vi "CSS validation.vi"() -> ()   [LabVIEW 2014]
uses:
  <vilib>/Utility/file.llb/Read From Spreadsheet File (string).vi
  <vilib>/Utility/file.llb/Write To Spreadsheet File (string).vi
panel:
  in  "cluster centers":string[](array[string])=["1 0 -1 1 -1 0 -4 1 -4 0 1", "2 0 -1 2 -1 0 -2 2 -2 0 2", "3 0 -3 3 -3 0 -2 3 -2 0 3", "4 0 -3 4 -3 0 -4 4 -4 0 4", "-1 1 -4 0 -4 4 -3 4 -4 0 -4 1 -1", "-1 2 -2 0 -2 3 -3 3 -2 0 -2 2 -1", "-4 1 -1 0 -1 2 -2 2 -1 0 -1 1 -4", "-4 4 -3 0 -3 3 -2 3 -3 0 -3 4 -4", "0 -4 1 -1 0 -3 3 -2 3 -3 0 -1 1 -4 0", "0 -4 4 -3 0 -1 2 -2 2 -1 0 -3 4 -4 0"]
  in  "cluster centers (original) 4":string[](array[string])=["0 -1 1 -4 0 -4 1 -1 0", "0 -1 2 -2 0 -2 2 -1 0", "0 -2 3 -3 0 -3 3 -2 0", "0 -3 4 -4 0 -4 4 -3 0", "0 -1 1 -4 4 -3 0 -3 4 -4 1 -1 0", "0 -1 2 -2 3 -3 0 -3 3 -2 2 -1 0", "0 -4 1 -1 2 -2 0 -2 2 -1 1 -4 0", "0 -4 4 -3 3 -2 0 -2 3 -3 4 -4 0", "0 -1 1 -4 0 -2 3 -3 0 -3 3 -2 0 -4 1 -1 0", "0 -1 2 -2 0 -4 4 -3 0 -3 4 -4 0 -2 2 -1 0"]
  in  "cluster centers 3":string[](array[string])=["0 -1 1 0 1 -4 0 -4 1 0 1 -1 0 -1 1 0 1 -4 0 -4 1 0 1 -1 0 -1 1 0 1 -4 0 -4 1 0 1 -1 0", "0 -1 2 0 2 -2 0 -2 2 0 2 -1 0 -1 2 0 2 -2 0 -2 2 0 2 -1 0 -1 2 0 2 -2 0 -2 2 0 2 -1 0", "0 -2 3 0 3 -3 0 -3 3 0 3 -2 0 -2 3 0 3 -3 0 -3 3 0 3 -2 0 -2 3 0 3 -3 0 -3 3 0 3 -2 0", "0 -3 4 0 4 -4 0 -4 4 0 4 -3 0 -3 4 0 4 -4 0 -4 4 0 4 -3 0 -3 4 0 4 -4 0 -4 4 0 4 -3 0", "0 -1 1 -4 0 -4 4 -3 0 -3 4 -4 0 -4 1 -1 0 0 -1 1 -4 0 -4 4 -3 0 -3 4 -4 0 -4 1 -1 0 0 -1 1 -4 0 -4 4 -3 0 -3 4 -4 0 -4 1 -1 0", "0 -1 2 -2 0 -2 3 -3 0 -3 3 -2 0 -2 2 -1 0 0 -1 2 -2 0 -2 3 -3 0 -3 3 -2 0 -2 2 -1 0 0 -1 2 -2 0 -2 3 -3 0 -3 3 -2 0 -2 2 -1 0", "0 -4 1 -1 0 -1 2 -2 0 -2 2 -1 0 -1 1 -4 0 0 -4 1 -1 0 -1 2 -2 0 -2 2 -1 0 -1 1 -4 0 0 -4 1 -1 0 -1 2 -2 0 -2 2 -1 0 -1 1 -4 0", "0 -4 4 -3 0 -3 3 -2 0 -2 3 -3 0 -3 4 -4 0 0 -4 4 -3 0 -3 3 -2 0 -2 3 -3 0 -3 4 -4 0 0 -4 4 -3 0 -3 3 -2 0 -2 3 -3 0 -3 4 -4 0", "0 -1 1 -4 0 -4 1 -1 0 -3 3 -2 0 -2 3 -3 0 -1 1 -4 0 -4 1 -1 0 -3 3 -2 0 -2 3 -3 0 -1 1 -4 0 -4 1 -1 0 -3 3 -2 0 -2 3 -3 0", "0 -4 4 -3 0 -3 4 -4 0 -2 2 -1 0 -1 2 -2 0 -4 4 -3 0 -3 4 -4 0 -2 2 -1 0 -1 2 -2 0 -4 4 -3 0 -3 4 -4 0 -2 2 -1 0 -1 2 -2 0"]
  out "size(s)":i32
  in  "cluster centers (original) 3":string[](array[string])=["0 -1 1 -4 0 -4 1 -1 0 -1 1 -4 0 -4 1 -1 0 -1 1 -4 0 -4 1 -1 0", "0 -1 2 -2 0 -2 2 -1 0 -1 2 -2 0 -2 2 -1 0 -1 2 -2 0 -2 2 -1 0", "0 -2 3 -3 0 -3 3 -2 0 -2 3 -3 0 -3 3 -2 0 -2 3 -3 0 -3 3 -2 0", "0 -3 4 -4 0 -4 4 -3 0 -3 4 -4 0 -4 4 -3 0 -3 4 -4 0 -4 4 -3 0", "0 -1 1 -4 4 -3 0 -3 4 -4 1 -1 0 -1 1 -4 4 -3 0 -3 4 -4 1 -1 0 -1 1 -4 4 -3 0 -3 4 -4 1 -1 0", "0 -1 2 -2 3 -3 0 -3 3 -2 2 -1 0 -1 2 -2 3 -3 0 -3 3 -2 2 -1 0 -1 2 -2 3 -3 0 -3 3 -2 2 -1 0", "0 -4 1 -1 2 -2 0 -2 2 -1 1 -4 0 -4 1 -1 2 -2 0 -2 2 -1 1 -4 0 -4 1 -1 2 -2 0 -2 2 -1 1 -4 0", "0 -4 4 -3 3 -2 0 -2 3 -3 4 -4 0 -4 4 -3 3 -2 0 -2 3 -3 4 -4 0 -4 4 -3 3 -2 0 -2 3 -3 4 -4 0", "0 -1 1 -4 0 -2 3 -3 0 -3 3 -2 0 -4 1 -1 0 -1 1 -4 0 -2 3 -3 0 -3 3 -2 0 -4 1 -1 0 -1 1 -4 0 -2 3 -3 0 -3 3 -2 0 -4 1 -1 0", "0 -1 2 -2 0 -4 4 -3 0 -3 4 -4 0 -2 2 -1 0 -1 2 -2 0 -4 4 -3 0 -3 4 -4 0 -2 2 -1 0 -1 2 -2 0 -4 4 -3 0 -3 4 -4 0 -2 2 -1 0"]
  in  "cluster centers (original) 2":string[](array[string])=["0 -1 1 -4 0 -4 1 -1 0", "0 -1 2 -2 0 -2 2 -1 0", "0 -2 3 -3 0 -3 3 -2 0", "0 -3 4 -4 0 -4 4 -3 0", "0 -1 1 -4 4 -3 0 -3 4 -4 1 -1 0", "0 -1 2 -2 3 -3 0 -3 3 -2 2 -1 0", "0 -4 1 -1 2 -2 0 -2 2 -1 1 -4 0", "0 -4 4 -3 3 -2 0 -2 3 -3 4 -4 0", "0 -1 1 -4 0 -2 3 -3 0 -3 3 -2 0 -4 1 -1 0", "0 -1 2 -2 0 -4 4 -3 0 -3 4 -4 0 -2 2 -1 0"]
  out "results":string[][](array[string])
  in  "cluster centers 2 centers for diagonals - long - original clusters 5":string[](array[string])=["1 0 -1 1 -1 0 -4 1 -4 0 1 0 -1 1 -1 0 -4 1 -4 0 1 0 -1 1 -1 0 -4 1 -4 0 1 0 -1 1 -1 0 -4 1 -4 0 1 0 -1 1 -1 0 -4 1 -4 0 1", "2 0 -1 2 -1 0 -2 2 -2 0 2 0 -1 2 -1 0 -2 2 -2 0 2 0 -1 2 -1 0 -2 2 -2 0 2 0 -1 2 -1 0 -2 2 -2 0 2 0 -1 2 -1 0 -2 2 -2 0 2", "3 0 -3 3 -3 0 -2 3 -2 0 3 0 -3 3 -3 0 -2 3 -2 0 3 0 -3 3 -3 0 -2 3 -2 0 3 0 -3 3 -3 0 -2 3 -2 0 3 0 -3 3 -3 0 -2 3 -2 0 3", "4 0 -3 4 -3 0 -4 4 -4 0 4 0 -3 4 -3 0 -4 4 -4 0 4 0 -3 4 -3 0 -4 4 -4 0 4 0 -3 4 -3 0 -4 4 -4 0 4 0 -3 4 -3 0 -4 4 -4 0 4", "-1 1 -4 0 -4 4 -3 4 -4 0 -4 1 -1 1 -4 0 -4 4 -3 4 -4 0 -4 1 -1 1 -4 0 -4 4 -3 4 -4 0 -4 1 -1 1 -4 0 -4 4 -3 4 -4 0 -4 1 -1 1 -4 0 -4 4 -3 4 -4 0 -4 1 -1", "-1 2 -2 0 -2 3 -3 3 -2 0 -2 2 -1 2 -2 0 -2 3 -3 3 -2 0 -2 2 -1 2 -2 0 -2 3 -3 3 -2 0 -2 2 -1 2 -2 0 -2 3 -3 3 -2 0 -2 2 -1 2 -2 0 -2 3 -3 3 -2 0 -2 2 -1", "-4 1 -1 0 -1 2 -2 2 -1 0 -1 1 -4 1 -1 0 -1 2 -2 2 -1 0 -1 1 -4 1 -1 0 -1 2 -2 2 -1 0 -1 1 -4 1 -1 0 -1 2 -2 2 -1 0 -1 1 -4 1 -1 0 -1 2 -2 2 -1 0 -1 1 -4", "-4 4 -3 0 -3 3 -2 3 -3 0 -3 4 -4 4 -3 0 -3 3 -2 3 -3 0 -3 4 -4 4 -3 0 -3 3 -2 3 -3 0 -3 4 -4 4 -3 0 -3 3 -2 3 -3 0 -3 4 -4 4 -3 0 -3 3 -2 3 -3 0 -3 4 -4", "0 1 -1 0 -3 3 0 3 -3 0 -1 1 0 1 -1 0 -3 3 0 3 -3 0 -1 1 0 1 -1 0 -3 3 0 3 -3 0 -1 1 0 1 -1 0 -3 3 0 3 -3 0 -1 1 0 1 -1 0 -3 3 0 3 -3 0 -1 1 0", "0 1 -4 0 -2 3 0 3 -2 0 -4 1 0 1 -4 0 -2 3 0 3 -2 0 -4 1 0 1 -4 0 -2 3 0 3 -2 0 -4 1 0 1 -4 0 -2 3 0 3 -2 0 -4 1 0 1 -4 0 -2 3 0 3 -2 0 -4 1 0", "0 4 -3 0 -1 2 0 2 -1 0 -3 4 0 4 -3 0 -1 2 0 2 -1 0 -3 4 0 4 -3 0 -1 2 0 2 -1 0 -3 4 0 4 -3 0 -1 2 0 2 -1 0 -3 4 0 4 -3 0 -1 2 0 2 -1 0 -3 4 0", "0 4 -4 0 -2 2 0 2 -2 0 -4 4 0 4 -4 0 -2 2 0 2 -2 0 -4 4 0 4 -4 0 -2 2 0 2 -2 0 -4 4 0 4 -4 0 -2 2 0 2 -2 0 -4 4 0 4 -4 0 -2 2 0 2 -2 0 -4 4 0"]
  in  "cluster centers 2 centers for diagonals - long - original clusters 4":string[](array[string])=["1 0 -1 1 -1 0 -4 1 -4 0 1 0 -1 1 -1 0 -4 1 -4 0 1 0 -1 1 -1 0 -4 1 -4 0 1 0 -1 1 -1 0 -4 1 -4 0 1", "2 0 -1 2 -1 0 -2 2 -2 0 2 0 -1 2 -1 0 -2 2 -2 0 2 0 -1 2 -1 0 -2 2 -2 0 2 0 -1 2 -1 0 -2 2 -2 0 2", "3 0 -3 3 -3 0 -2 3 -2 0 3 0 -3 3 -3 0 -2 3 -2 0 3 0 -3 3 -3 0 -2 3 -2 0 3 0 -3 3 -3 0 -2 3 -2 0 3", "4 0 -3 4 -3 0 -4 4 -4 0 4 0 -3 4 -3 0 -4 4 -4 0 4 0 -3 4 -3 0 -4 4 -4 0 4 0 -3 4 -3 0 -4 4 -4 0 4", "-1 1 -4 0 -4 4 -3 4 -4 0 -4 1 -1 1 -4 0 -4 4 -3 4 -4 0 -4 1 -1 1 -4 0 -4 4 -3 4 -4 0 -4 1 -1 1 -4 0 -4 4 -3 4 -4 0 -4 1 -1", "-1 2 -2 0 -2 3 -3 3 -2 0 -2 2 -1 2 -2 0 -2 3 -3 3 -2 0 -2 2 -1 2 -2 0 -2 3 -3 3 -2 0 -2 2 -1 2 -2 0 -2 3 -3 3 -2 0 -2 2 -1", "-4 1 -1 0 -1 2 -2 2 -1 0 -1 1 -4 1 -1 0 -1 2 -2 2 -1 0 -1 1 -4 1 -1 0 -1 2 -2 2 -1 0 -1 1 -4 1 -1 0 -1 2 -2 2 -1 0 -1 1 -4", "-4 4 -3 0 -3 3 -2 3 -3 0 -3 4 -4 4 -3 0 -3 3 -2 3 -3 0 -3 4 -4 4 -3 0 -3 3 -2 3 -3 0 -3 4 -4 4 -3 0 -3 3 -2 3 -3 0 -3 4 -4", "0 1 -1 0 -3 3 0 3 -3 0 -1 1 0 1 -1 0 -3 3 0 3 -3 0 -1 1 0 1 -1 0 -3 3 0 3 -3 0 -1 1 0 1 -1 0 -3 3 0 3 -3 0 -1 1 0", "0 1 -4 0 -2 3 0 3 -2 0 -4 1 0 1 -4 0 -2 3 0 3 -2 0 -4 1 0 1 -4 0 -2 3 0 3 -2 0 -4 1 0 1 -4 0 -2 3 0 3 -2 0 -4 1 0", "0 4 -3 0 -1 2 0 2 -1 0 -3 4 0 4 -3 0 -1 2 0 2 -1 0 -3 4 0 4 -3 0 -1 2 0 2 -1 0 -3 4 0 4 -3 0 -1 2 0 2 -1 0 -3 4 0", "0 4 -4 0 -2 2 0 2 -2 0 -4 4 0 4 -4 0 -2 2 0 2 -2 0 -4 4 0 4 -4 0 -2 2 0 2 -2 0 -4 4 0 4 -4 0 -2 2 0 2 -2 0 -4 4 0"]
  in  "cluster centers 2 centers for diagonals - long - original clusters 3":string[](array[string])=["1 0 -1 1 -1 0 -4 1 -4 0 1 0 -1 1 -1 0 -4 1 -4 0 1 0 -1 1 -1 0 -4 1 -4 0 1", "2 0 -1 2 -1 0 -2 2 -2 0 2 0 -1 2 -1 0 -2 2 -2 0 2 0 -1 2 -1 0 -2 2 -2 0 2", "3 0 -3 3 -3 0 -2 3 -2 0 3 0 -3 3 -3 0 -2 3 -2 0 3 0 -3 3 -3 0 -2 3 -2 0 3", "4 0 -3 4 -3 0 -4 4 -4 0 4 0 -3 4 -3 0 -4 4 -4 0 4 0 -3 4 -3 0 -4 4 -4 0 4", "-1 1 -4 0 -4 4 -3 4 -4 0 -4 1 -1 1 -4 0 -4 4 -3 4 -4 0 -4 1 -1 1 -4 0 -4 4 -3 4 -4 0 -4 1 -1", "-1 2 -2 0 -2 3 -3 3 -2 0 -2 2 -1 2 -2 0 -2 3 -3 3 -2 0 -2 2 -1 2 -2 0 -2 3 -3 3 -2 0 -2 2 -1", "-4 1 -1 0 -1 2 -2 2 -1 0 -1 1 -4 1 -1 0 -1 2 -2 2 -1 0 -1 1 -4 1 -1 0 -1 2 -2 2 -1 0 -1 1 -4", "-4 4 -3 0 -3 3 -2 3 -3 0 -3 4 -4 4 -3 0 -3 3 -2 3 -3 0 -3 4 -4 4 -3 0 -3 3 -2 3 -3 0 -3 4 -4", "0 1 -1 0 -3 3 0 3 -3 0 -1 1 0 1 -1 0 -3 3 0 3 -3 0 -1 1 0 1 -1 0 -3 3 0 3 -3 0 -1 1 0", "0 1 -4 0 -2 3 0 3 -2 0 -4 1 0 1 -4 0 -2 3 0 3 -2 0 -4 1 0 1 -4 0 -2 3 0 3 -2 0 -4 1 0", "0 4 -3 0 -1 2 0 2 -1 0 -3 4 0 4 -3 0 -1 2 0 2 -1 0 -3 4 0 4 -3 0 -1 2 0 2 -1 0 -3 4 0", "0 4 -4 0 -2 2 0 2 -2 0 -4 4 0 4 -4 0 -2 2 0 2 -2 0 -4 4 0 4 -4 0 -2 2 0 2 -2 0 -4 4 0"]
  in  "cluster centers 2 centers for diagonals - short - original clusters":string[](array[string])=["1 0 -1 1 -1 0 -4 1 -4 0 1", "2 0 -1 2 -1 0 -2 2 -2 0 2", "3 0 -3 3 -3 0 -2 3 -2 0 3", "4 0 -3 4 -3 0 -4 4 -4 0 4", "-1 1 -4 0 -4 4 -3 4 -4 0 -4 1 -1", "-1 2 -2 0 -2 3 -3 3 -2 0 -2 2 -1", "-4 1 -1 0 -1 2 -2 2 -1 0 -1 1 -4", "-4 4 -3 0 -3 3 -2 3 -3 0 -3 4 -4", "0 1 -1 0 -3 3 0 3 -3 0 -1 1 0", "0 1 -4 0 -2 3 0 3 -2 0 -4 1 0", "0 4 -3 0 -1 2 0 2 -1 0 -3 4 0", "0 4 -4 0 -2 2 0 2 -2 0 -4 4 0"]
  in  "cluster centers 2 centers for diagonals - long - original clusters":string[](array[string])=["1 0 -1 1 -1 0 -4 1 -4 0 1 0 -1 1 -1 0 -4 1 -4 0 1", "2 0 -1 2 -1 0 -2 2 -2 0 2 0 -1 2 -1 0 -2 2 -2 0 2", "3 0 -3 3 -3 0 -2 3 -2 0 3 0 -3 3 -3 0 -2 3 -2 0 3", "4 0 -3 4 -3 0 -4 4 -4 0 4 0 -3 4 -3 0 -4 4 -4 0 4", "-1 1 -4 0 -4 4 -3 4 -4 0 -4 1 -1 1 -4 0 -4 4 -3 4 -4 0 -4 1 -1", "-1 2 -2 0 -2 3 -3 3 -2 0 -2 2 -1 2 -2 0 -2 3 -3 3 -2 0 -2 2 -1", "-4 1 -1 0 -1 2 -2 2 -1 0 -1 1 -4 1 -1 0 -1 2 -2 2 -1 0 -1 1 -4", "-4 4 -3 0 -3 3 -2 3 -3 0 -3 4 -4 4 -3 0 -3 3 -2 3 -3 0 -3 4 -4", "0 1 -1 0 -3 3 0 3 -3 0 -1 1 0 1 -1 0 -3 3 0 3 -3 0 -1 1 0", "0 1 -4 0 -2 3 0 3 -2 0 -4 1 0 1 -4 0 -2 3 0 3 -2 0 -4 1 0", "0 4 -3 0 -1 2 0 2 -1 0 -3 4 0 4 -3 0 -1 2 0 2 -1 0 -3 4 0", "0 4 -4 0 -2 2 0 2 -2 0 -4 4 0 4 -4 0 -2 2 0 2 -2 0 -4 4 0"]
  in  "cluster centers (original) long 5":string[](array[string])=["1 0 -1 1 -1 0 -4 1 -4 0 1 0 -1 1 -1 0 -4 1 -4 0 1 0 -1 1 -1 0 -4 1 -4 0 1 0 -1 1 -1 0 -4 1 -4 0 1 0 -1 1 -1 0 -4 1 -4 0 1", "2 0 -1 2 -1 0 -2 2 -2 0 2 0 -1 2 -1 0 -2 2 -2 0 2 0 -1 2 -1 0 -2 2 -2 0 2 0 -1 2 -1 0 -2 2 -2 0 2 0 -1 2 -1 0 -2 2 -2 0 2", "3 0 -3 3 -3 0 -2 3 -2 0 3 0 -3 3 -3 0 -2 3 -2 0 3 0 -3 3 -3 0 -2 3 -2 0 3 0 -3 3 -3 0 -2 3 -2 0 3 0 -3 3 -3 0 -2 3 -2 0 3", "4 0 -3 4 -3 0 -4 4 -4 0 4 0 -3 4 -3 0 -4 4 -4 0 4 0 -3 4 -3 0 -4 4 -4 0 4 0 -3 4 -3 0 -4 4 -4 0 4 0 -3 4 -3 0 -4 4 -4 0 4", "-1 1 -4 0 -4 4 -3 4 -4 0 -4 1 -1 1 -4 0 -4 4 -3 4 -4 0 -4 1 -1 1 -4 0 -4 4 -3 4 -4 0 -4 1 -1 1 -4 0 -4 4 -3 4 -4 0 -4 1 -1 1 -4 0 -4 4 -3 4 -4 0 -4 1 -1", "-1 2 -2 0 -2 3 -3 3 -2 0 -2 2 -1 2 -2 0 -2 3 -3 3 -2 0 -2 2 -1 2 -2 0 -2 3 -3 3 -2 0 -2 2 -1 2 -2 0 -2 3 -3 3 -2 0 -2 2 -1 2 -2 0 -2 3 -3 3 -2 0 -2 2 -1", "-4 1 -1 0 -1 2 -2 2 -1 0 -1 1 -4 1 -1 0 -1 2 -2 2 -1 0 -1 1 -4 1 -1 0 -1 2 -2 2 -1 0 -1 1 -4 1 -1 0 -1 2 -2 2 -1 0 -1 1 -4 1 -1 0 -1 2 -2 2 -1 0 -1 1 -4", "-4 4 -3 0 -3 3 -2 3 -3 0 -3 4 -4 4 -3 0 -3 3 -2 3 -3 0 -3 4 -4 4 -3 0 -3 3 -2 3 -3 0 -3 4 -4 4 -3 0 -3 3 -2 3 -3 0 -3 4 -4 4 -3 0 -3 3 -2 3 -3 0 -3 4 -4", "0 -4 1 -1 0 -3 3 -2 3 -3 0 -1 1 -4 0 -4 1 -1 0 -3 3 -2 3 -3 0 -1 1 -4 0 -4 1 -1 0 -3 3 -2 3 -3 0 -1 1 -4 0 -4 1 -1 0 -3 3 -2 3 -3 0 -1 1 -4 0 -4 1 -1 0 -3 3 -2 3 -3 0 -1 1 -4 0", "0 -4 4 -3 0 -1 2 -2 2 -1 0 -3 4 -4 0 -4 4 -3 0 -1 2 -2 2 -1 0 -3 4 -4 0 -4 4 -3 0 -1 2 -2 2 -1 0 -3 4 -4 0 -4 4 -3 0 -1 2 -2 2 -1 0 -3 4 -4 0 -4 4 -3 0 -1 2 -2 2 -1 0 -3 4 -4 0"]
  in  "cluster centers (original) long 4":string[](array[string])=["1 0 -1 1 -1 0 -4 1 -4 0 1 0 -1 1 -1 0 -4 1 -4 0 1 0 -1 1 -1 0 -4 1 -4 0 1 0 -1 1 -1 0 -4 1 -4 0 1", "2 0 -1 2 -1 0 -2 2 -2 0 2 0 -1 2 -1 0 -2 2 -2 0 2 0 -1 2 -1 0 -2 2 -2 0 2 0 -1 2 -1 0 -2 2 -2 0 2", "3 0 -3 3 -3 0 -2 3 -2 0 3 0 -3 3 -3 0 -2 3 -2 0 3 0 -3 3 -3 0 -2 3 -2 0 3 0 -3 3 -3 0 -2 3 -2 0 3", "4 0 -3 4 -3 0 -4 4 -4 0 4 0 -3 4 -3 0 -4 4 -4 0 4 0 -3 4 -3 0 -4 4 -4 0 4 0 -3 4 -3 0 -4 4 -4 0 4", "-1 1 -4 0 -4 4 -3 4 -4 0 -4 1 -1 1 -4 0 -4 4 -3 4 -4 0 -4 1 -1 1 -4 0 -4 4 -3 4 -4 0 -4 1 -1 1 -4 0 -4 4 -3 4 -4 0 -4 1 -1", "-1 2 -2 0 -2 3 -3 3 -2 0 -2 2 -1 2 -2 0 -2 3 -3 3 -2 0 -2 2 -1 2 -2 0 -2 3 -3 3 -2 0 -2 2 -1 2 -2 0 -2 3 -3 3 -2 0 -2 2 -1", "-4 1 -1 0 -1 2 -2 2 -1 0 -1 1 -4 1 -1 0 -1 2 -2 2 -1 0 -1 1 -4 1 -1 0 -1 2 -2 2 -1 0 -1 1 -4 1 -1 0 -1 2 -2 2 -1 0 -1 1 -4", "-4 4 -3 0 -3 3 -2 3 -3 0 -3 4 -4 4 -3 0 -3 3 -2 3 -3 0 -3 4 -4 4 -3 0 -3 3 -2 3 -3 0 -3 4 -4 4 -3 0 -3 3 -2 3 -3 0 -3 4 -4", "0 -4 1 -1 0 -3 3 -2 3 -3 0 -1 1 -4 0 -4 1 -1 0 -3 3 -2 3 -3 0 -1 1 -4 0 -4 1 -1 0 -3 3 -2 3 -3 0 -1 1 -4 0 -4 1 -1 0 -3 3 -2 3 -3 0 -1 1 -4 0", "0 -4 4 -3 0 -1 2 -2 2 -1 0 -3 4 -4 0 -4 4 -3 0 -1 2 -2 2 -1 0 -3 4 -4 0 -4 4 -3 0 -1 2 -2 2 -1 0 -3 4 -4 0 -4 4 -3 0 -1 2 -2 2 -1 0 -3 4 -4 0"]
  in  "cluster centers (original) long 3":string[](array[string])=["1 0 -1 1 -1 0 -4 1 -4 0 1 0 -1 1 -1 0 -4 1 -4 0 1 0 -1 1 -1 0 -4 1 -4 0 1", "2 0 -1 2 -1 0 -2 2 -2 0 2 0 -1 2 -1 0 -2 2 -2 0 2 0 -1 2 -1 0 -2 2 -2 0 2", "3 0 -3 3 -3 0 -2 3 -2 0 3 0 -3 3 -3 0 -2 3 -2 0 3 0 -3 3 -3 0 -2 3 -2 0 3", "4 0 -3 4 -3 0 -4 4 -4 0 4 0 -3 4 -3 0 -4 4 -4 0 4 0 -3 4 -3 0 -4 4 -4 0 4", "-1 1 -4 0 -4 4 -3 4 -4 0 -4 1 -1 1 -4 0 -4 4 -3 4 -4 0 -4 1 -1 1 -4 0 -4 4 -3 4 -4 0 -4 1 -1", "-1 2 -2 0 -2 3 -3 3 -2 0 -2 2 -1 2 -2 0 -2 3 -3 3 -2 0 -2 2 -1 2 -2 0 -2 3 -3 3 -2 0 -2 2 -1", "-4 1 -1 0 -1 2 -2 2 -1 0 -1 1 -4 1 -1 0 -1 2 -2 2 -1 0 -1 1 -4 1 -1 0 -1 2 -2 2 -1 0 -1 1 -4", "-4 4 -3 0 -3 3 -2 3 -3 0 -3 4 -4 4 -3 0 -3 3 -2 3 -3 0 -3 4 -4 4 -3 0 -3 3 -2 3 -3 0 -3 4 -4", "0 -4 1 -1 0 -3 3 -2 3 -3 0 -1 1 -4 0 -4 1 -1 0 -3 3 -2 3 -3 0 -1 1 -4 0 -4 1 -1 0 -3 3 -2 3 -3 0 -1 1 -4 0", "0 -4 4 -3 0 -1 2 -2 2 -1 0 -3 4 -4 0 -4 4 -3 0 -1 2 -2 2 -1 0 -3 4 -4 0 -4 4 -3 0 -1 2 -2 2 -1 0 -3 4 -4 0"]
  in  "cluster centers 2 long":string[](array[string])=["0 1 0 -1 1 0 1 -1 0 -4 1 0 1 -4 0 1 0 -1 1 0 1 -1 0 -4 1 0 1 -4 0", "0 2 0 -1 2 0 2 -1 0 -2 2 0 2 -2 0 2 0 -1 2 0 2 -1 0 -2 2 0 2 -2 0", "0 3 0 -3 3 0 3 -3 0 -2 3 0 3 -2 0 3 0 -3 3 0 3 -3 0 -2 3 0 3 -2 0", "0 4 0 -3 4 0 4 -3 0 -4 4 0 4 -4 0 4 0 -3 4 0 4 -3 0 -4 4 0 4 -4 0", "0 -1 1 -4 0 -4 4 -3 4 -4 0 -4 1 -1 0 -1 1 -4 0 -4 4 -3 4 -4 0 -4 1 -1 0", "0 -1 2 -2 0 -2 3 -3 3 -2 0 -2 2 -1 0 -1 2 -2 0 -2 3 -3 3 -2 0 -2 2 -1 0", "0 -4 1 -1 0 -1 2 -2 2 -1 0 -1 1 -4 0 -4 1 -1 0 -1 2 -2 2 -1 0 -1 1 -4 0", "0 -4 4 -3 0 -3 3 -2 3 -3 0 -3 4 -4 0 -4 4 -3 0 -3 3 -2 3 -3 0 -3 4 -4 0", "0 -4 1 -1 0 -3 3 -2 3 -3 0 -1 1 -4 0 -4 1 -1 0 -3 3 -2 3 -3 0 -1 1 -4 0", "0 -4 4 -3 0 -1 2 -2 2 -1 0 -3 4 -4 0 -4 4 -3 0 -1 2 -2 2 -1 0 -3 4 -4 0"]
  in  "cluster centers (original) long":string[](array[string])=["1 0 -1 1 -1 0 -4 1 -4 0 1 0 -1 1 -1 0 -4 1 -4 0 1", "2 0 -1 2 -1 0 -2 2 -2 0 2 0 -1 2 -1 0 -2 2 -2 0 2", "3 0 -3 3 -3 0 -2 3 -2 0 3 0 -3 3 -3 0 -2 3 -2 0 3", "4 0 -3 4 -3 0 -4 4 -4 0 4 0 -3 4 -3 0 -4 4 -4 0 4", "-1 1 -4 0 -4 4 -3 4 -4 0 -4 1 -1 1 -4 0 -4 4 -3 4 -4 0 -4 1 -1", "-1 2 -2 0 -2 3 -3 3 -2 0 -2 2 -1 2 -2 0 -2 3 -3 3 -2 0 -2 2 -1", "-4 1 -1 0 -1 2 -2 2 -1 0 -1 1 -4 1 -1 0 -1 2 -2 2 -1 0 -1 1 -4", "-4 4 -3 0 -3 3 -2 3 -3 0 -3 4 -4 4 -3 0 -3 3 -2 3 -3 0 -3 4 -4", "0 -4 1 -1 0 -3 3 -2 3 -3 0 -1 1 -4 0 -4 1 -1 0 -3 3 -2 3 -3 0 -1 1 -4 0", "0 -4 4 -3 0 -1 2 -2 2 -1 0 -3 4 -4 0 -4 4 -3 0 -1 2 -2 2 -1 0 -3 4 -4 0"]
  in  "cluster centers 2 centers for diagonals":string[](array[string])=["0 1 0 -1 1 0 1 -1 0 -4 1 0 1 -4 0", "0 2 0 -1 2 0 2 -1 0 -2 2 0 2 -2 0", "0 3 0 -3 3 0 3 -3 0 -2 3 0 3 -2 0", "0 4 0 -3 4 0 4 -3 0 -4 4 0 4 -4 0", "0 -1 1 -4 0 -4 4 -3 4 -4 0 -4 1 -1 0", "0 -1 2 -2 0 -2 3 -3 3 -2 0 -2 2 -1 0", "0 -4 1 -1 0 -1 2 -2 2 -1 0 -1 1 -4 0", "0 -4 4 -3 0 -3 3 -2 3 -3 0 -3 4 -4 0", "0 1 -1 0 -3 3 0 3 -3 0 -1 1 0", "0 1 -4 0 -2 3 0 3 -2 0 -4 1 0", "0 4 -3 0 -1 2 0 2 -1 0 -3 4 0", "0 4 -4 0 -2 2 0 2 -2 0 -4 4 0"]
  in  "cluster centers 2 centers for diagonals - long clusters  with zero side clusters":string[](array[string])=["0 1 0 -1 1 0 1 -1 0 -4 1 0 1 -4 0 1 0 -1 1 0 1 -1 0 -4 1 0 1 -4 0", "0 2 0 -1 2 0 2 -1 0 -2 2 0 2 -2 0 2 0 -1 2 0 2 -1 0 -2 2 0 2 -2 0", "0 3 0 -3 3 0 3 -3 0 -2 3 0 3 -2 0 3 0 -3 3 0 3 -3 0 -2 3 0 3 -2 0", "0 4 0 -3 4 0 4 -3 0 -4 4 0 4 -4 0 4 0 -3 4 0 4 -3 0 -4 4 0 4 -4 0", "0 -1 1 -4 0 -4 4 -3 4 -4 0 -4 1 -1 0 -1 1 -4 0 -4 4 -3 4 -4 0 -4 1 -1 0", "0 -1 2 -2 0 -2 3 -3 3 -2 0 -2 2 -1 0 -1 2 -2 0 -2 3 -3 3 -2 0 -2 2 -1 0", "0 -4 1 -1 0 -1 2 -2 2 -1 0 -1 1 -4 0 -4 1 -1 0 -1 2 -2 2 -1 0 -1 1 -4 0", "0 -4 4 -3 0 -3 3 -2 3 -3 0 -3 4 -4 0 -4 4 -3 0 -3 3 -2 3 -3 0 -3 4 -4 0", "0 1 -1 0 -3 3 0 3 -3 0 -1 1 0 1 -1 0 -3 3 0 3 -3 0 -1 1 0", "0 1 -4 0 -2 3 0 3 -2 0 -4 1 0 1 -4 0 -2 3 0 3 -2 0 -4 1 0", "0 4 -3 0 -1 2 0 2 -1 0 -3 4 0 4 -3 0 -1 2 0 2 -1 0 -3 4 0", "0 4 -4 0 -2 2 0 2 -2 0 -4 4 0 4 -4 0 -2 2 0 2 -2 0 -4 4 0"]
  in  "cluster centers 2":string[](array[string])=["0 1 0 -1 1 0 1 -1 0 -4 1 0 1 -4 0", "0 2 0 -1 2 0 2 -1 0 -2 2 0 2 -2 0", "0 3 0 -3 3 0 3 -3 0 -2 3 0 3 -2 0", "0 4 0 -3 4 0 4 -3 0 -4 4 0 4 -4 0", "0 -1 1 -4 0 -4 4 -3 4 -4 0 -4 1 -1 0", "0 -1 2 -2 0 -2 3 -3 3 -2 0 -2 2 -1 0", "0 -4 1 -1 0 -1 2 -2 2 -1 0 -1 1 -4 0", "0 -4 4 -3 0 -3 3 -2 3 -3 0 -3 4 -4 0", "0 -4 1 -1 0 -3 3 -2 3 -3 0 -1 1 -4 0", "0 -4 4 -3 0 -1 2 -2 2 -1 0 -3 4 -4 0"]
  out "appended array 2":string[][](array[string])
  in  "file path (dialog if empty)":path
  in  "cluster centers (original)":string[](array[string])=["1 0 -1 1 -1 0 -4 1 -4 0 1", "2 0 -1 2 -1 0 -2 2 -2 0 2", "3 0 -3 3 -3 0 -2 3 -2 0 3", "4 0 -3 4 -3 0 -4 4 -4 0 4", "-1 1 -4 0 -4 4 -3 4 -4 0 -4 1 -1", "-1 2 -2 0 -2 3 -3 3 -2 0 -2 2 -1", "-4 1 -1 0 -1 2 -2 2 -1 0 -1 1 -4", "-4 4 -3 0 -3 3 -2 3 -3 0 -3 4 -4", "0 -4 1 -1 0 -3 3 -2 3 -3 0 -1 1 -4 0", "0 -4 4 -3 0 -1 2 -2 2 -1 0 -3 4 -4 0"]
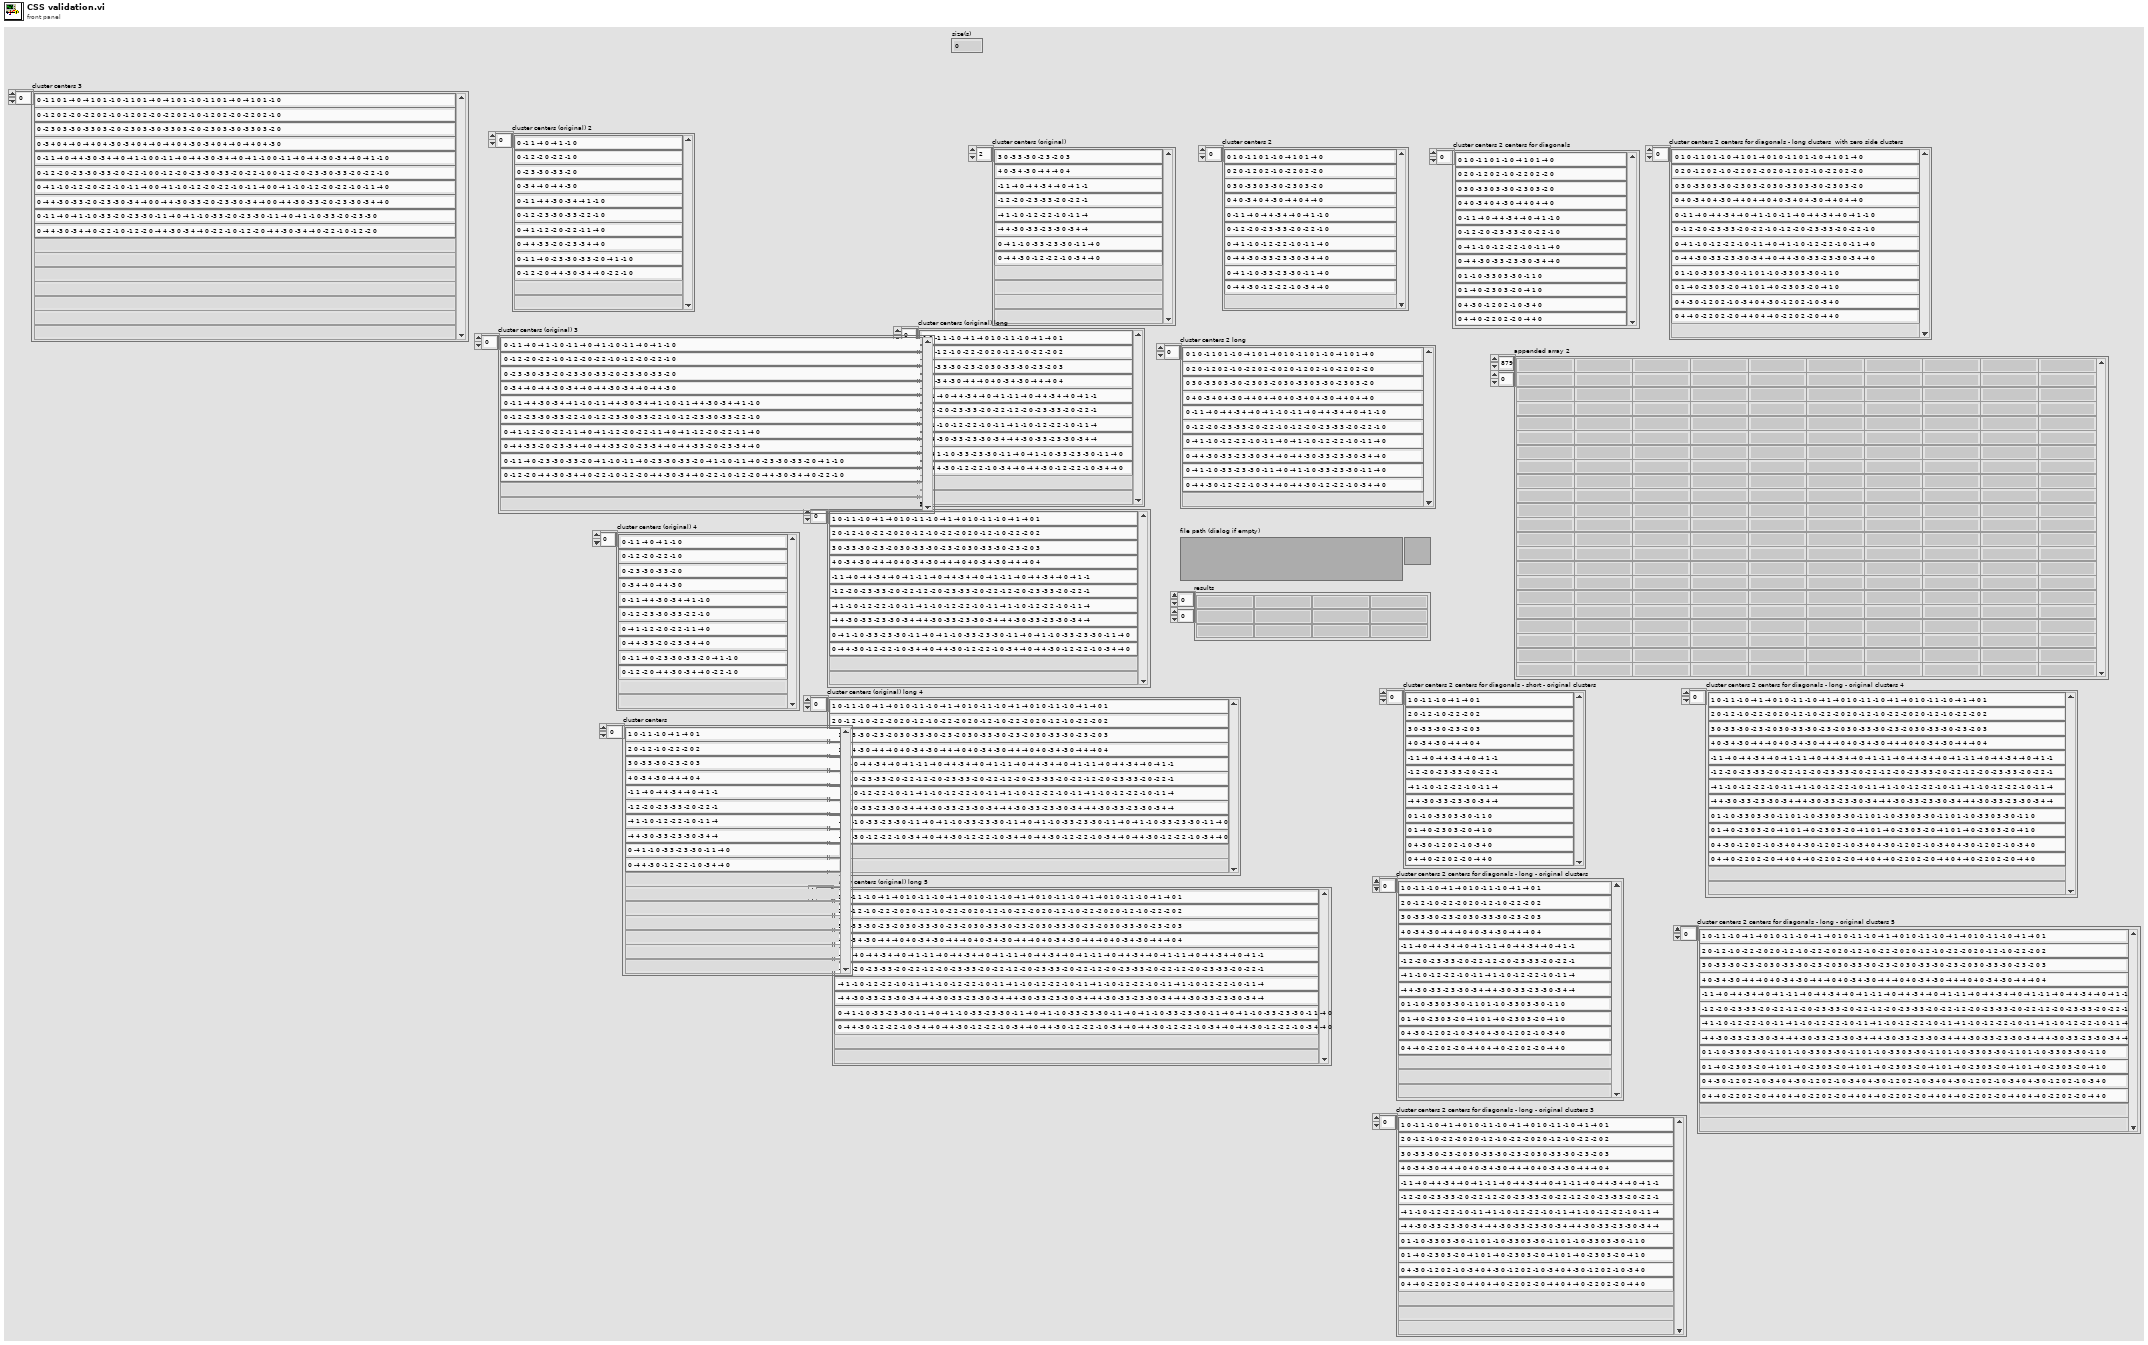
[diagram p1: front panel]
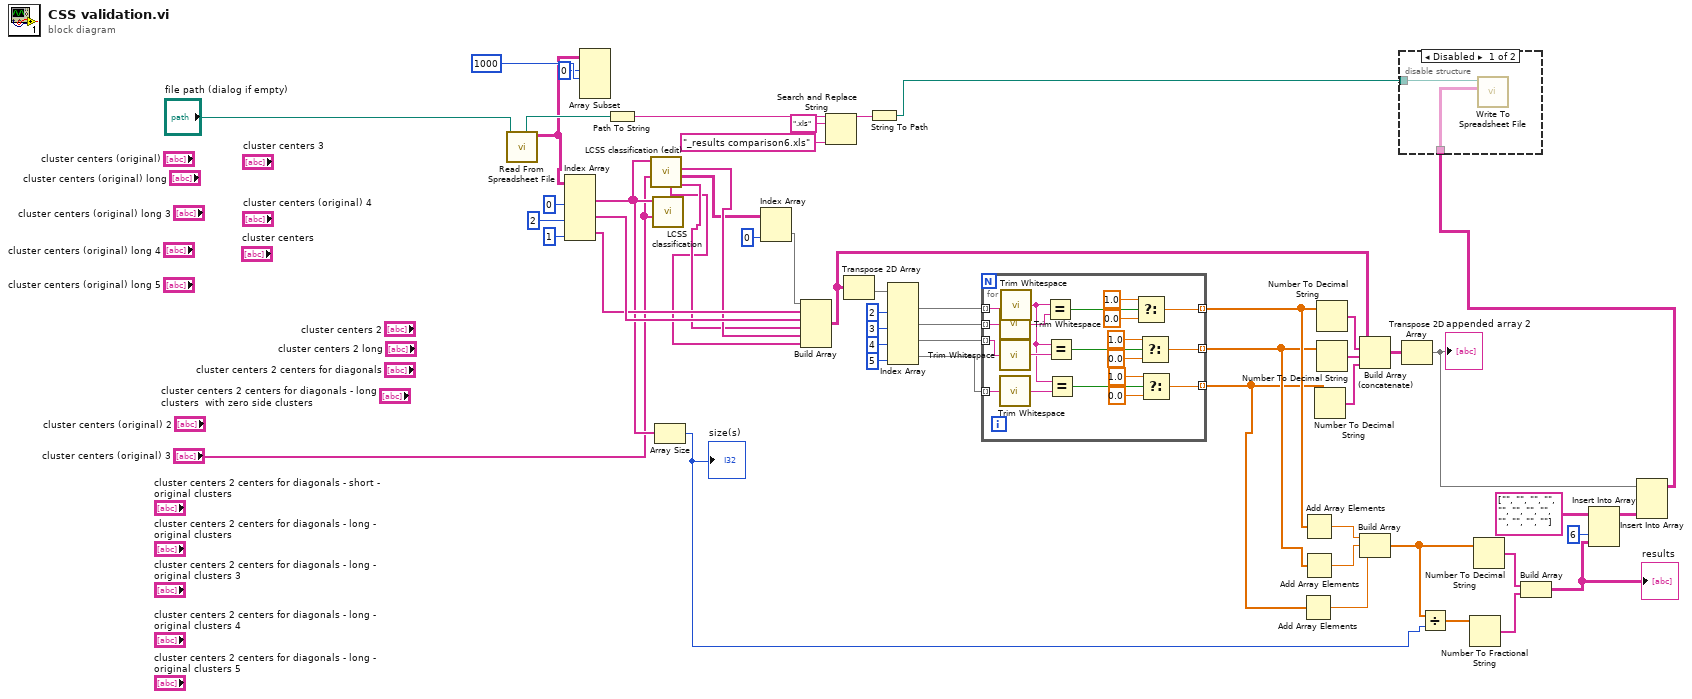
[diagram p0: block diagram]
diagram:
  n1 = call-poly <vilib>:"Read From Spreadsheet File.vi"("file path (dialog if empty)"="file path (dialog if empty)") -> ("all rows"=w6:string[][], "new file path (Not A Path if cancelled)"=w50:path)  [unwired: 6 in, 3 out]
  n2 = Index Array(array=w6, index (col) #1=0 ("disabled index (col)"), index (col) #2=2 ("index (col)"), index (col) #3=1 ("index (col)")) -> (element #1=w7:string[], element #2=w32:string[], element #3=w30:string[])  [unwired: 3 in]
  n3 = Array Subset(array=w6, index (row)=0 ("index"), length (row)=1000 ("index")) -> ()  [unwired: 2 in, 1 out]
  n4 = Path To String(path=w50) -> (string=w49:string)
  n5 = call "LCSS classification (edit).vi"("cluster centers"="cluster centers (original) 3", "Patterns in"=w7) -> ("Assigned cluster (0) unassigned"=w3:string[], "patterns in, distance values"=w4:string[][], "Assigned cluster 2nd method"=w5:string[], "Assigned cluster 3rd method 2"=w2:string[])  [unwired: 5 in, 1 out]
  n6 = call "LCSS classification.vi"("cluster centers"="cluster centers (original) 3", "Patterns in"=w7) -> ()  [unwired: 5 in, 5 out]
  n7 = Array Size(array=w7) -> (size(s)=w10:i32)
  "size(s)" <- w10
  n8 = Index Array(array=w4, index (col)=0 ("disabled index (col)")) -> (element=w53:string[])  [unwired: 1 in]
  n9 = Build Array(w53, w30, w32, w3, w5, w2) -> (w34:string[][])
  n10 = Search and Replace String(input string=w49, search string=".xls", replace string="_results comparison6.xls" ("replace string (\"\")")) -> (result string=w46:string)  [unwired: 5 in, 3 out]
  n11 = Transpose 2D Array(2D array=w34) -> (transposed array=w37:string[][])
  n12 = String To Path(string=w46) -> (path=w45:path)
  n13 = Index Array(array=w37, index (col) #1=2 ("disabled index (col)"), index (col) #2=3 ("index (col)"), index (col) #3=4 ("index (col)"), index (col) #4=5 ("index (col)")) -> (element #1=w40:string[], element #2=w39:string[], element #3=w38:string[], element #4=w28:string[])  [unwired: 4 in]
  n14 = for {
    tunnel: w40 -> [w66] mode=indexing
    tunnel: w39 -> [w65] mode=indexing
    tunnel: w38 -> [w64] mode=indexing
    tunnel: [w68] -> w15 mode=indexing
    tunnel: [w67] -> w14 mode=indexing
    tunnel: w28 -> [w59] mode=indexing
    tunnel: [w55] -> w13 mode=indexing
    n15 = call <vilib>:"Trim Whitespace.vi"("string"=w65) -> ("trimmed string"=w63:string)  [unwired: 1 in]
    n16 = call <vilib>:"Trim Whitespace.vi"("string"=w64) -> ("trimmed string"=w62:string)  [unwired: 1 in]
    n17 = call <vilib>:"Trim Whitespace.vi"("string"=w59) -> ("trimmed string"=w61:string)  [unwired: 1 in]
    n18 = call <vilib>:"Trim Whitespace.vi"("string"=w66) -> ("trimmed string"=w60:string)  [unwired: 1 in]
    n19 = Equal?(x=w60, y=w63) -> (x = y?=w74:bool)
    n20 = Equal?(x=w60, y=w62) -> (x = y?=w69:bool)
    n21 = Equal?(x=w60, y=w61) -> (x = y?=w56:bool)
    n22 = Select(t=1.0, s=w74, f=0.0) -> (s? t:f=w68:dbl)
    n23 = Select(t=1.0, s=w69, f=0.0) -> (s? t:f=w67:dbl)
    n24 = Select(t=1.0, s=w56, f=0.0) -> (s? t:f=w55:dbl)
  }
  n25 = Add Array Elements(numeric array=w13) -> (sum=w18:dbl)
  n26 = Add Array Elements(numeric array=w15) -> (sum=w16:dbl)
  n27 = Add Array Elements(numeric array=w14) -> (sum=w17:dbl)
  n28 = Number To Decimal String(number=w13) -> (decimal integer string=w27:string[])  [unwired: 1 in]
  n29 = Number To Decimal String(number=w15) -> (decimal integer string=w36:string[])  [unwired: 1 in]
  n30 = Number To Decimal String(number=w14) -> (decimal integer string=w35:string[])  [unwired: 1 in]
  n31 = Build Array (concatenate)(w34, w36, w35, w27) -> (w33:string[][])
  n32 = Build Array(w16, w17, w18) -> (w19:dbl[])
  n33 = Transpose 2D Array(2D array=w33) -> (transposed array=w12:string[][])
  "appended array 2" <- w12
  n34 = Divide(x=w19, y=w10) -> (x/y=w20:dbl[])
  n35 = Number To Fractional String(number=w20) -> (F-format string=w22:string[])  [unwired: 3 in]
  n36 = Number To Decimal String(number=w19) -> (decimal integer string=w21:string[])  [unwired: 1 in]
  n37 = Build Array(w21, w22) -> (w26:string[][])
  "results" <- w26
  n38 = Insert Into Array(array=string[][] [["", "", "", "", "", ""], ["", "", "", "", "", ""]] ("appended array 3"), index (col)=6 ("disabled index (col)"), new element=w26) -> (w25:string[][])  [unwired: 1 in]
  n39 = Insert Into Array(array=w12, new element=w25) -> (w11:string[][])  [unwired: 2 in]
  n40 = disable-structure shown="Disabled" {
    disable-tunnel: w45 -> [w76 _]
    disable-tunnel: w11 -> [w75 _]
    frame Disabled {
      n41 = call-poly <vilib>:"Write To Spreadsheet File.vi"("2D data"=w75, "file path (dialog if empty)"=w76) -> ()  [unwired: 6 in, 1 out]
    }
    frame Enabled {
    }
  }
